vi "grid_distance.vi"(1 "x":dbl) -> (0 "distance_mm":dbl)   [LabVIEW 2017]
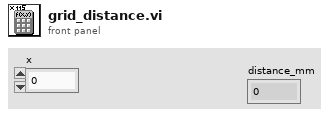
[diagram p1: front panel]
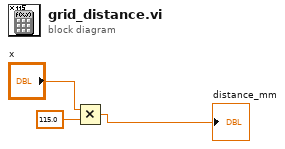
[diagram p0: block diagram]
diagram:
  n1 = Multiply(x="x", y=115.0) -> (x*y=→"distance_mm":dbl)
